vi "SwissSPAD Live_Update Image Information Event.vi"(8 "error in (no error)":errorcluster, 10 "Calling VI Name":string, 11 "User Event in":refnum<user-event>) -> ()   [LabVIEW 2021]
uses:
  SwissSPAD Live_Settings Event.ctl
  SwissSPAD Live_Settings Window Messages.ctl
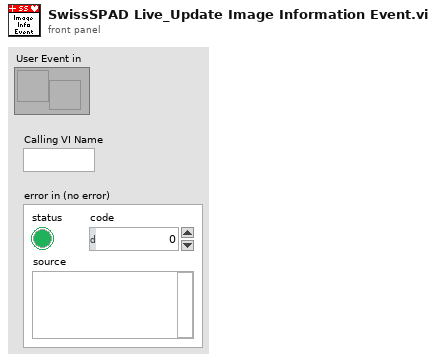
[diagram p1: front panel]
types:
  T1 = typedef "SwissSPAD Live_Settings Window Messages.ctl" = enum16{"Idle", "Subscribe", "Unsubscribe", "Refresh Parameter", "Refresh All Parameters", "Quit"}
  T2 = typedef "SwissSPAD Live_Settings Event.ctl" = cluster{"Settings Message":T1, "Sender":string, "Control Label":string, "Data":variant}
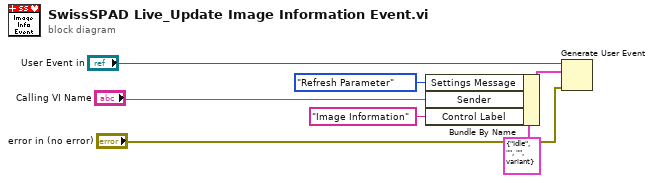
[diagram p0: block diagram]
diagram:
  n1 = Bundle By Name(cluster=T2 {"Settings Message"=enum."Idle", "Sender"="", "Control Label"="", "Data"=variant} ("Settings Event"), "Settings Message"=SwissSPAD_Live_Settings_Window_Messages."Refresh Parameter", "Sender"="Calling VI Name", "Control Label"="Image Information") -> (w5:T2)
  n2 = Generate User Event(user event="User Event in", event data cluster=w5, error in="error in (no error)") -> ()  [unwired: 1 in, 2 out]
